vi "Get Value by Array (String).vi"(8 "error in (no error)":errorcluster, 10 "Keys":string[](array[string]), 11 "JSON Object in":refnum<class "JSON Helper.lvclass">) -> (0 "error out":errorcluster, 2 "JSON out":refnum<class "JSON Helper.lvclass">)   [LabVIEW 2016]
uses:
  JSON Helper/JSON Helper.lvclass
  JSON Helper/To More Specific Type (String).vi
  JSON Datatype/JSON Null.lvclass
  JSON String/JSON String.lvclass
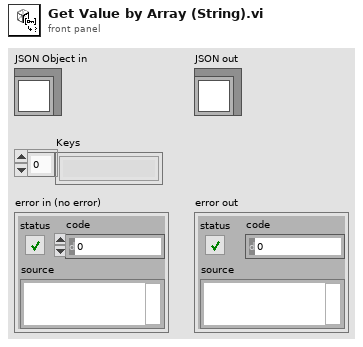
[diagram p1: front panel]
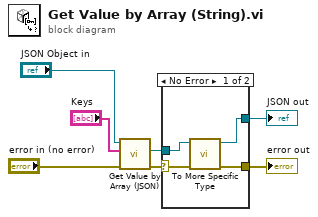
[diagram p0: block diagram]
diagram:
  n1 = call "Get Value by Array (JSON).vi"("error in (no error)"="error in (no error)", "Keys"="Keys", "JSON in"="JSON Object in") -> ("error out"=w4:errorcluster, "JSON out"=w3:refnum<class "JSON Helper.lvclass">)  [unwired: 7 in]
  n2 = case shown="No Error" w4 {
    selector: w4 -> [w11 w12]
    tunnel: w3 -> [w10 _]
    tunnel: [w9 _] -> w2
    tunnel: [w8 w12] -> w1
    frame No Error {
      n3 = call-poly "To More Specific Type.vi"("error in (no error)"=w11, "JSON Datatype in"=w10) -> ("error out"=w8:errorcluster, "JSON Datatype out"=w9:refnum<class "JSON String.lvclass">)  [unwired: 8 in]
    }
    frame Error {
    }
  }
  "JSON out" <- w2
  "error out" <- w1
